vi "word finder.vi"(6 "time out":u16=4, 8 "error in":errorcluster, 9 "delay":u32=50, 10 "expresion":string, 11 "reference":refnum<visa-resource-name>) -> (0 "error out":errorcluster, 1 "bad state?":bool, 2 "response":string, 3 "reference out":refnum<visa-resource-name>)   [LabVIEW 2021]
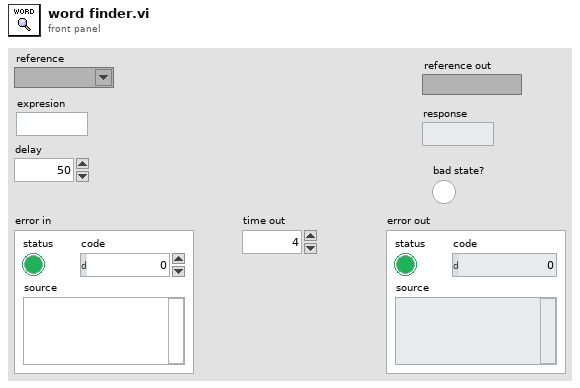
[diagram p1: front panel]
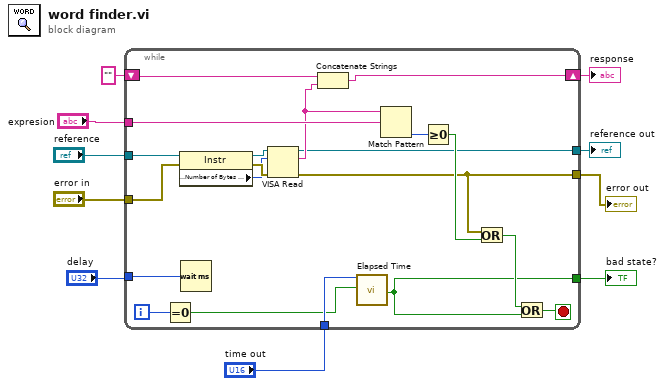
[diagram p0: block diagram]
diagram:
  n1 = while {
    tunnel: "reference" -> [w25]
    tunnel: "expresion" -> [w24]
    shift-right: [w22] -> w7
    shift-left: "" -> [w23]
    tunnel: [w20] -> w6
    tunnel: "delay" -> [w19]
    tunnel: [w18] -> w3
    tunnel: "error in" -> [w17]
    tunnel: "time out" -> [w16]
    tunnel: [w13] -> w1
    i -> [w12]
    stop <- w15 stop-if-true
    n2 = Equal To 0?(x=w12) -> (x = 0?=w11:bool)
    n3 = property class="Instr"(reference=w25, error in=w17) -> (reference out=w28:refnum<visa-resource-name>, error out=w27:errorcluster, "Serial Settings:Number of Bytes at Serial Port"=w26:u32)
    n4 = Wait (ms)(milliseconds to wait=w19) -> ()  [unwired: 1 out]
    n5 = VISA Read(VISA resource name=w28, byte count=w26, error in (no error)=w27) -> (VISA resource name out=w20:refnum<visa-resource-name>, read buffer=w21:string, error out=w18:errorcluster)  [unwired: 1 out]
    n6 = Concatenate Strings(w23, w21) -> (w22:string)
    n7 = call "Elapsed Time"("Time Target (s)"=w16, "Reset"=w11) -> ("Time has Elapsed"=w13:bool)  [unwired: 10 in, 7 out]
    n8 = Match Pattern(string=w21, regular expression=w24) -> (offset past match=w30:i32)  [unwired: 1 in, 3 out]
    n9 = Greater Or Equal To 0?(x=w30) -> (x >= 0?=w29:bool)
    n10 = Or(x=w18, y=w29) -> (x .or. y?=w14:bool)
    n11 = Or(x=w14, y=w13) -> (x .or. y?=w15:bool)
  }
  "response" <- w7
  "reference out" <- w6
  "error out" <- w3
  "bad state?" <- w1
